vi "Master Setup Auto Correct.vi"(9 "Master File Path":path, 10 "Current File Paths (in)":path[](array[path]), 11 "Setup Patterns":string[](array[string])) -> (2 "Current File Paths (out)":path[](array[path]))   [LabVIEW 2017]
panel:
  out "Actual Setup Patterns":string[](array[string])
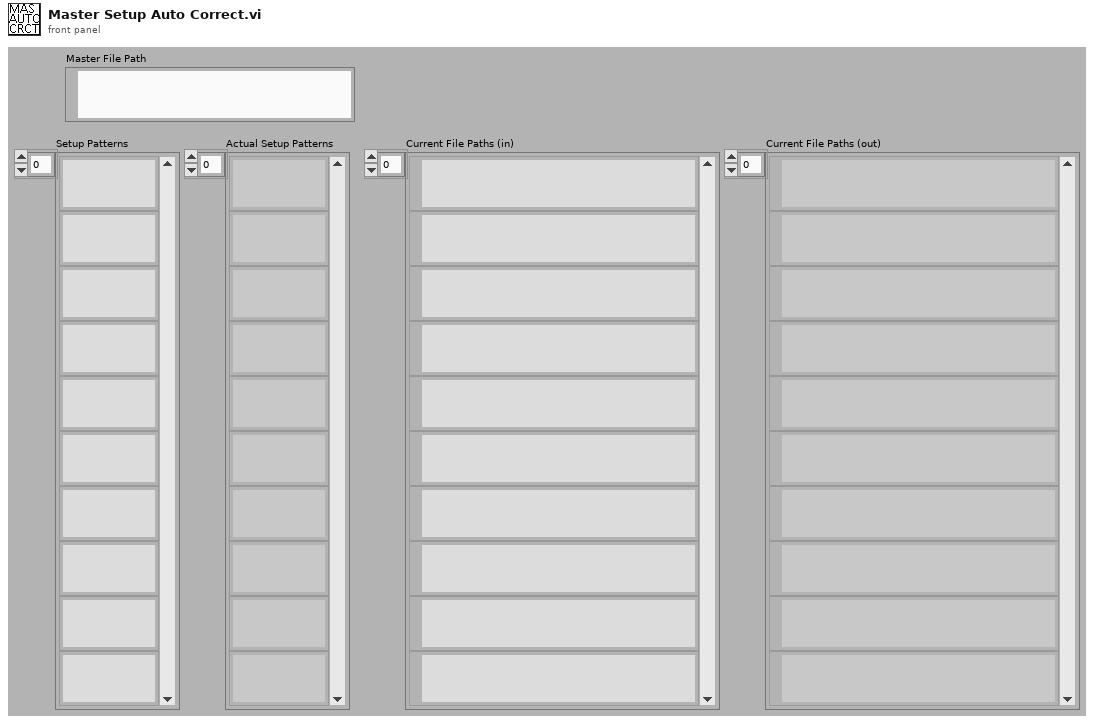
[diagram p1: front panel]
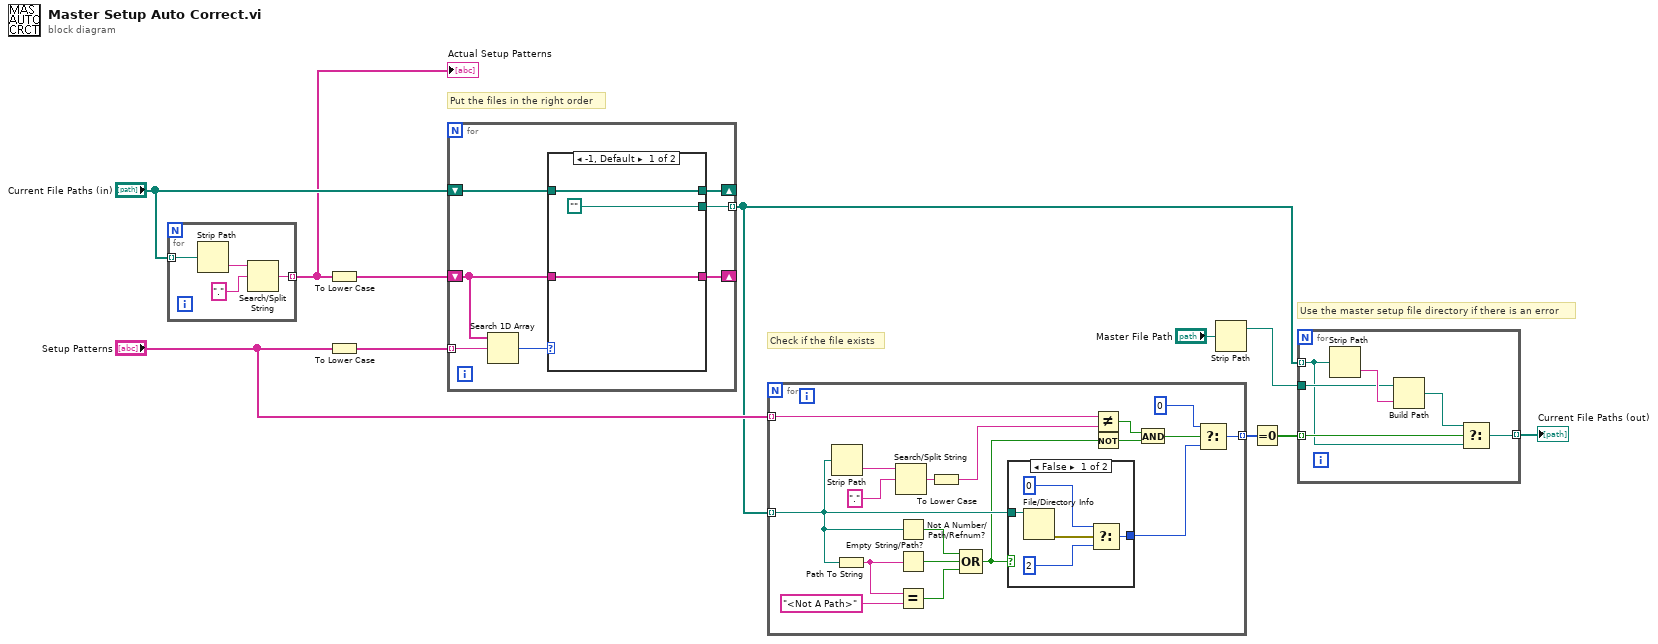
[diagram p0: block diagram]
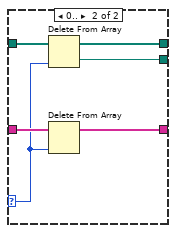
[diagram p2: hidden frame]
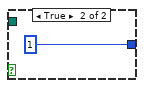
[diagram p3: hidden frame]
diagram:
  # "Use the master setup file directory if there is an error"
  # "Check if the file exists"
  # "Put the files in the right order"
  n1 = for {
    tunnel: "Current File Paths (in)" -> [w15] mode=indexing
    tunnel: [w12] -> w3 mode=indexing
    n2 = Strip Path(path=w15) -> (name=w13:string)  [unwired: 1 out]
    n3 = Search/Split String(string=w13, search string/char (-)=".") -> (match + rest of string=w12:string)  [unwired: 1 in, 2 out]
  }
  "Actual Setup Patterns" <- w3
  n4 = To Lower Case(string=w3) -> (all lower case string=w2:string[])
  n5 = To Lower Case(string="Setup Patterns") -> (all lower case string=w1:string[])
  n6 = for {
    tunnel: w1 -> [w22] mode=indexing
    shift-right: [w20] -> _
    shift-left: "Current File Paths (in)" -> [w21]
    shift-right: [w17] -> _
    shift-left: w2 -> [w18]
    tunnel: [w16] -> w4 mode=indexing
    n7 = Search 1D Array(1D array=w18, element=w22) -> (index of element=w19:i32)  [unwired: 1 in]
    n8 = case shown="-1, Default" w19 {
      selector: w19 -> [_ w27]
      tunnel: w21 -> [w24 w29]
      tunnel: [w24 w28] -> w20
      tunnel: w18 -> [w25 w31]
      tunnel: [w25 w30] -> w17
      tunnel: [path "" w26] -> w16
      frame -1, Default {
      }
      frame 0.. {
        n9 = Delete From Array(array=w29, index=w27) -> (deleted portion=w26:path, array with subset deleted=w28:path[])  [unwired: 1 in]
        n10 = Delete From Array(array=w31, index=w27) -> (array with subset deleted=w30:string[])  [unwired: 1 in, 1 out]
      }
    }
  }
  n11 = for {
    tunnel: w4 -> [w44] mode=indexing
    tunnel: [w39] -> w8 mode=indexing
    tunnel: "Setup Patterns" -> [w32] mode=indexing
    n12 = Strip Path(path=w44) -> (name=w43:string)  [unwired: 1 out]
    n13 = Path To String(path=w44) -> (string=w47:string)
    n14 = Search/Split String(string=w43, search string/char (-)=".") -> (match + rest of string=w38:string)  [unwired: 1 in, 2 out]
    n15 = Not A Number/Path/Refnum?(number/path/refnum=w44) -> (NaN/Path/Refnum?=w48:bool)
    n16 = Empty String/Path?(string/path=w47) -> (empty?=w49:bool)
    n17 = Equal?(x=w47, y="<Not A Path>") -> (x = y?=w45:bool)
    n18 = To Lower Case(string=w38) -> (all lower case string=w33:string)
    n19 = Compound Arithmetic op=OR(w48, w49, w45) -> (w35:bool)
    n20 = case shown="False" w35 {
      tunnel: w44 -> [w54 _]
      tunnel: [w50 u16 1] -> w41
      frame False {
        n21 = File/Directory Info(path=w54) -> (error out=w53:errorcluster)  [unwired: 1 in, 6 out]
        n22 = Select(t=u16 0, s=w53, f=u16 2) -> (s? t:f=w50:u16)
      }
      frame True {
      }
    }
    n23 = Not Equal?(x=w32, y=w33) -> (x != y?=w36:bool)
    n24 = Not(x=w35) -> (.not. x?=w34:bool)
    n25 = And(x=w36, y=w34) -> (x .and. y?=w37:bool)
    n26 = Select(t=u16 0, s=w37, f=w41) -> (s? t:f=w39:u16)
  }
  n27 = Strip Path(path="Master File Path") -> (stripped path=w6:path)  [unwired: 1 out]
  n28 = Equal To 0?(x=w8) -> (x = 0?=w7:bool[])
  n29 = for {
    tunnel: w7 -> [w61] mode=indexing
    tunnel: w4 -> [w57] mode=indexing
    tunnel: w6 -> [w59]
    tunnel: [w56] -> w5 mode=indexing
    n30 = Strip Path(path=w57) -> (name=w60:string)  [unwired: 1 out]
    n31 = Build Path(base path=w59, name or relative path=w60) -> (appended path=w58:path)
    n32 = Select(t=w58, s=w61, f=w57) -> (s? t:f=w56:path)
  }
  "Current File Paths (out)" <- w5
